vi "Position Control.vi"(7 "theta":dbl, 8 "Y":dbl, 9 "X":dbl, 10 "Y0":dbl, 11 "X0":dbl) -> (2 "y out":dbl, 3 "x out":dbl)   [LabVIEW 2016]
uses:
  <vilib>/Analysis/coordinate.llb/2D Cartesian Coordinate Rotation (Scalar).vi
  <vilib>/addons/control/pid/pid.llb/PID (DBL Array).vi
  <vilib>/addons/control/pid/NI_PID_pid.lvlib
  <vilib>/Analysis/NI_AALPro.lvlib
panel:
  in  "reinitialize? (F)":bool
  out "dt out (s)":dbl format="%.3f"
  in  "output range":cluster{"output high":dbl, "output low":dbl}[](array[cluster])=[{"output high"=100.0, "output low"=-100.0}]
  in  "PID gains":T1(array[cluster])=[{"proportional gain (Kc)"=0.01, "integral time (Ti, min)"=0.01, "derivative time (Td, min)"=0.0}]
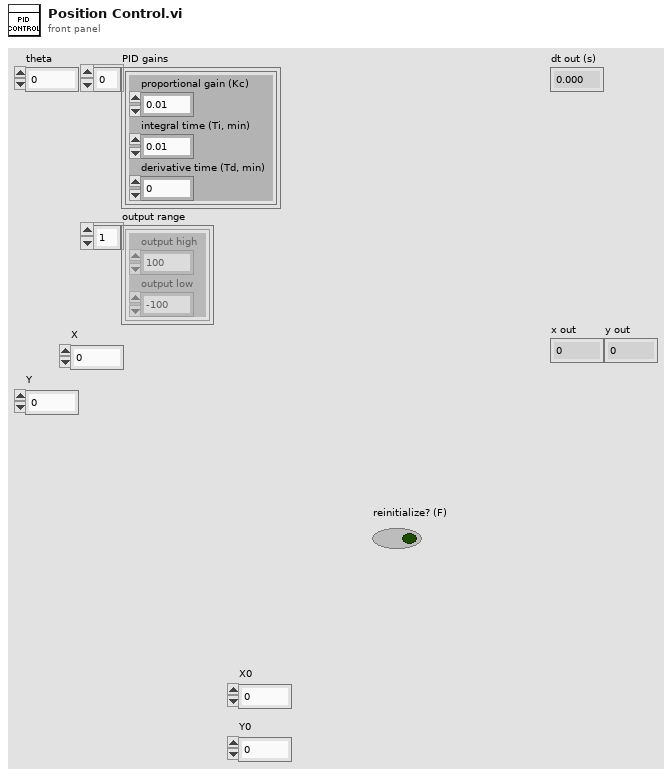
[diagram p1: front panel]
types:
  T1 = cluster{"proportional gain (Kc)":dbl, "integral time (Ti, min)":dbl, "derivative time (Td, min)":dbl}[]
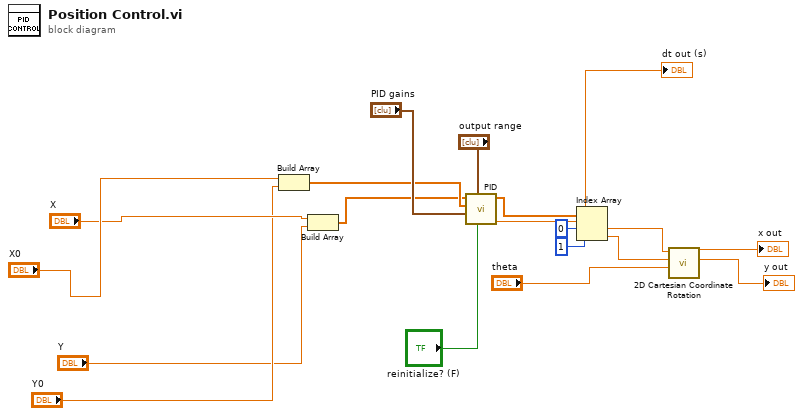
[diagram p0: block diagram]
diagram:
  n1 = Build Array("X0", "Y0") -> (w4:dbl[])
  n2 = Build Array("X", "Y") -> (w3:dbl[])
  n3 = call-poly <vilib>:"PID.vi"("reinitialize? (F)"="reinitialize? (F)", "output range"="output range", "PID gains"="PID gains", "process variable"=w4, "setpoint"=w3) -> ("dt out (s)"=→"dt out (s)":dbl, "output"=w13:dbl[])  [unwired: 5 in]
  n4 = Index Array(array=w13, index #1=0 ("index"), index #2=1 ("index")) -> (element #1=w11:dbl, element #2=w10:dbl)
  n5 = call-poly <vilib>:"2D Cartesian Coordinate Rotation.vi"("theta"="theta", "y"=w10, "x"=w11) -> ("y out"=→"y out":dbl, "x out"=→"x out":dbl)  [unwired: 6 in, 1 out]
